vi "ADIS16470 IMU Example.vi"() -> ()   [LabVIEW 2019]
uses:
  <vilib>/Utility/RT CPU Load.ctl
  ADIS16470Lib/Typedef/ADIS16470 Hardware Configuration.ctl
  <vilib>/Rock Robotics/WPI/SPI/WPI_SPIMode.ctl
  <vilib>/Rock Robotics/SystemInterfaces/DIO/FPGA_DIOChannel.ctl
  <vilib>/Rock Robotics/SystemInterfaces/spilib/spi_bus.ctl
  ADIS16470Lib/Typedef/ADIS16470 Calibration Time.ctl
  ADIS16470Lib/SubVI/ADIS16470 Globals.vi
  <vilib>/NI_Real-Time Target Support.lvlib
panel:
  out "DiagStat":u16
  out "TempDegC":dbl
  out "RegAccumData":dbl[](array[numeric])
  out "RawReadData":u16[](array[numeric])
  out "Loop State":i32
  in  "Use Register Read Mode":bool
  in  "Initial Calibration Time (4s)":T1=enum."4s"
  in  "Recalibrate?":bool
  in  "Reset?":bool
  out "Integrated Gyro Angle":T2(graph)
  out "Calibrated?":bool
  out "IMU Detected?":bool
  in  "Hardware Config":T3={"SPI Clock Rate (Hz)"=2000000.0, "IMU SPI Mode (3)"=enum."Mode 3 (Clk Idle High,Sample on Trailing)", "IMU Reset Pin"=enum."SPI Port CS2", "IMU SPI Bus"=enum."SPI On-Board, CS0", "IMU Data Ready Pin"=enum."SPI Port CS1", "Stall Config"={"Pow2BytesPerRead"=1, "StallTicks"=1000, "CsToSclkTicks"=5}}
  out "CPU loads":T7[](array[typedef]) {"ISR (%)" format="%#.2f"; "Idle (%)" format="%#.2f"; "Background (%)" format="%#.2f"; "Normal (%)" format="%#.2f"; "Above Normal (%)" format="%#.2f"; "High (%)" format="%#.2g"; "Timed Structures (%)" format="%#.2g"; "Time Critical (%)" format="%#.2g"; "Total (%)" format="%#.2g"}
  in  "stop":bool
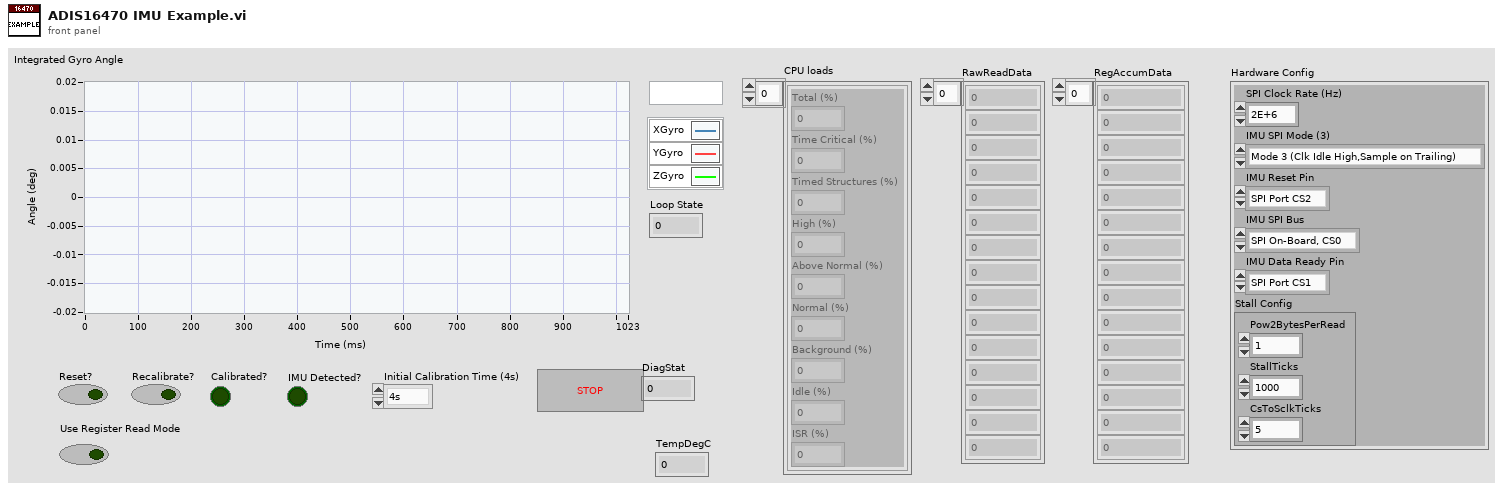
[diagram p1: front panel]
types:
  T1 = typedef "ADIS16470 Calibration Time.ctl" = enum16{"32ms", "64ms", "128ms", "256ms", "512ms", "1s", "2s", "4s", "8s", "16s", "32s", "64s"}
  T2 = cluster{"XAngle":dbl, "YAngle":dbl, "ZAngle":dbl}
  T3 = typedef "ADIS16470 Hardware Configuration.ctl" = cluster{"SPI Clock Rate (Hz)":dbl, "IMU SPI Mode (3)":T4, "IMU Reset Pin":T5, "IMU SPI Bus":T6, "IMU Data Ready Pin":T5, "Stall Config":cluster{"Pow2BytesPerRead":u8, "StallTicks":u16, "CsToSclkTicks":u8}}
  T4 = typedef "WPI_SPIMode.ctl" = enum16{"Mode 0 (Clk Idle Low,Sample on Leading)", "Mode 1 (Clk Idle Low,Sample on Trailing)", "Mode 2 (Clk Idle High,Sample on Leading)", "Mode 3 (Clk Idle High,Sample on Trailing)"}
  T5 = typedef "FPGA_DIOChannel.ctl" = enum8{"DIO 0", "DIO 1", "DIO 2", "DIO 3", "DIO 4", "DIO 5", "DIO 6", "DIO 7", "DIO 8", "DIO 9", "DIO MXP 0", "DIO MXP 1", "DIO MXP 2", "DIO MXP 3", "DIO MXP 4", "DIO MXP 5", "DIO MXP 6", "DIO MXP 7", "DIO MXP 8", "DIO MXP 9", "DIO MXP 10", "DIO MXP 11", "DIO MXP 12", "DIO MXP 13", "DIO MXP 14", "DIO MXP 15", "SPI Port CS1", "SPI Port CS2", "SPI Port CS3", "SPI Port MISO", "SPI Port MOSI", "Invalid"}
  T6 = typedef "spi_bus.ctl" = enum16{"SPI On-Board, CS0", "SPI On-Board, CS1", "SPI On-Board, CS2", "SPI On-Board, CS3", "SPI MXP", "Invalid"}
  T7 = typedef "NI_Real-Time Target Support.lvlib/RT CPU Load.ctl" = cluster{"Total (%)":dbl, "Time Critical (%)":dbl, "Timed Structures (%)":dbl, "High (%)":dbl, "Above Normal (%)":dbl, "Normal (%)":dbl, "Background (%)":dbl, "Idle (%)":dbl, "ISR (%)":dbl}
  T8 = typedef "ADIS16470 Device Reference.ctl" = cluster{"DevStatus":errorcluster, "Hardware Config":T3, "Calibration Complete":refnum<notifier>, "Status FIFO":refnum<k33>, "Last Value Reference":refnum<data-value>, "Sychronous Process VI":T9, "Cmd FIFO":refnum<k33>, "Source":T10, "Data FIFO":refnum<k33>, "Calibration Time":T1}
  T9 = typedef "ADIS16470 Process.ctl" = refnum<vi>
  T10 = typedef "FPGA_CounterEncoderSourceConvertionLVSourceType.ctl" = cluster{"DevStatus":errorcluster, "AnalogTriggerMode?":bool, "DigitalMode":cluster{"DIO Channel":T11}, "AnalogTriggerMode":cluster{"AnalogTriggerIndex":T12, "OutputType":T13}}
  T11 = typedef "FPGA_DIODigitalSourceChannel.ctl" = enum8{"DIO 0", "DIO 1", "DIO 2", "DIO 3", "DIO 4", "DIO 5", "DIO 6", "DIO 7", "DIO 8", "DIO 9", "DIO MXP 0", "DIO MXP 1", "DIO MXP 2", "DIO MXP 3", "DIO MXP 4", "DIO MXP 5", "DIO MXP 6", "DIO MXP 7", "DIO MXP 8", "DIO MXP 9", "DIO MXP 10", "DIO MXP 11", "DIO MXP 12", "DIO MXP 13", "DIO MXP 14", "DIO MXP 15", "SPI Port CS1", "SPI Port CS2", "SPI Port CS3", "SPI Port MISO", "SPI Port MOSI", "Disabled"}
  T12 = typedef "FPGA_AnalogTriggerIndex.ctl" = enum8{"Trig 0", "Trig 1", "Trig 2", "Trig 3", "Trig 4", "Trig 5", "Trig 6", "Trig 7", "Invalid"}
  T13 = typedef "FPGA_AnalogTriggerOutType.ctl" = enum16{"InWindow", "TriggerState", "Rising", "Falling"}
  T14 = typedef "ADIS16470 Status.ctl" = cluster{"Calibrated?":bool, "IMU Detected?":bool}
  T15 = typedef "ADIS16470 Data.ctl" = cluster{"XAngle":dbl, "YAngle":dbl, "ZAngle":dbl}
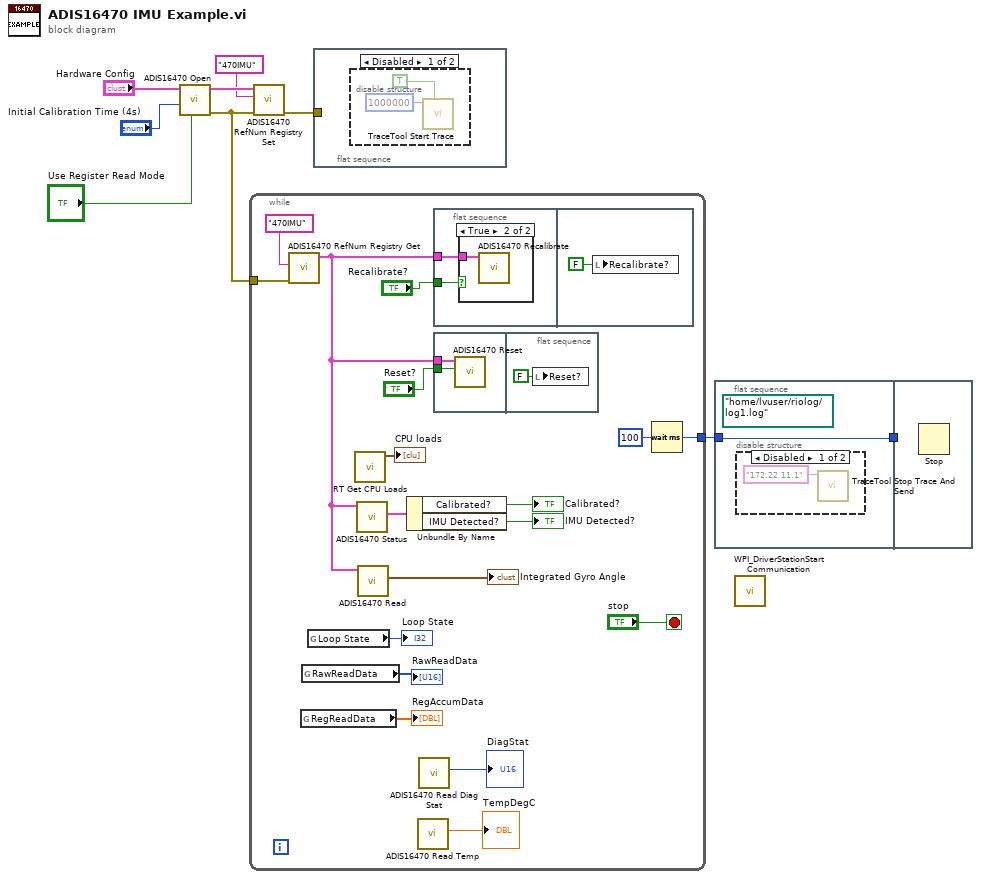
[diagram p0: block diagram]
diagram:
  n1 = call "ADIS16470 Open.vi"("Use Register Read Mode"="Use Register Read Mode", "Initial Calibration Time (4s)"="Initial Calibration Time (4s)", "Hardware Config"="Hardware Config") -> ("error out"=w2:errorcluster, "ADIS16470DevRef"=w4:T8)  [unwired: 7 in]
  n2 = while {
    tunnel: [w24] -> w9
    tunnel: w2 -> [w17]
    stop <- "stop" stop-if-true
    n3 = call "ADIS16470 RefNum Registry Get.vi"("error in (no error)"=w17, "refnum name"="470IMU") -> ("ADIS16470DevRef out"=w15:T8)  [unwired: 8 in, 1 out]
    n4 = global read "ADIS16470 Globals.vi" "RegReadData"() -> (→"RegAccumData":dbl[])
    n5 = global read "ADIS16470 Globals.vi" "RawReadData"() -> (→"RawReadData":u16[])
    n6 = global read "ADIS16470 Globals.vi" "Loop State"() -> (→"Loop State":i32)
    n7 = call <vilib>:"RT Get CPU Loads.vi"() -> ("CPU loads"=→"CPU loads":T7[])  [unwired: 10 in, 1 out]
    n8 = call "ADIS16470 Status.vi"("ADIS16470DevRef"=w15) -> ("ADIS16470 Status"=w22:T14)  [unwired: 8 in, 2 out]
    n9 = call "ADIS16470 Read.vi"("ADIS16470DevRef"=w15) -> ("ADIS16470 Value"=→"Integrated Gyro Angle":T15)  [unwired: 7 in, 3 out]
    n10 = Unbundle By Name(w22) -> ("Calibrated?"=→"Calibrated?":bool, "IMU Detected?"=→"IMU Detected?":bool)
    n11 = call "ADIS16470 Read Temp.vi"() -> ("TempDegC"=→"TempDegC":dbl)  [unwired: 9 in, 2 out]
    n12 = call "ADIS16470 Read Diag Stat.vi"() -> ("DiagStat"=→"DiagStat":u16)  [unwired: 9 in, 2 out]
    n13 = flat-sequence {
      tunnel: "Recalibrate?" -> [w28]
      tunnel: w15 -> [w29]
      frame #0 {
        n14 = case shown="True" w28 {
          tunnel: w29 -> [_ w30]
          frame False {
          }
          frame True {
            n15 = call "ADIS16470 Recalibrate.vi"("ADIS16470DevRef in"=w30) -> ()  [unwired: 9 in, 2 out]
          }
        }
      }
      frame #1 {
        n16 = local write "Recalibrate?"(FALSE ("Recalibrate?")) -> ()
      }
    }
    n17 = flat-sequence {
      tunnel: "Reset?" -> [w33]
      tunnel: w15 -> [w32]
      frame #0 {
        n18 = call "ADIS16470 Reset.vi"("Reset?"=w33, "ADIS16470DevRef"=w32) -> ()  [unwired: 8 in, 2 out]
      }
      frame #1 {
        n19 = local write "Reset?"(FALSE ("Reset?")) -> ()
      }
    }
    n20 = Wait (ms)(milliseconds to wait=u32 100) -> (millisecond timer value=w24:u32)
  }
  n21 = call "ADIS16470 RefNum Registry Set.vi"("error in (no error)"=w2, "refnum name"="470IMU", "ADIS16470DevRef in"=w4) -> ("error out"=w5:errorcluster)  [unwired: 7 in, 1 out]
  n22 = flat-sequence {
    tunnel: w5 -> [_]
    frame #0 {
      n23 = disable-structure shown="Disabled" {
        frame Disabled {
          n24 = call <vilib>:"TraceTool Start Trace.vi"("Detailed Tracing? (F)"=TRUE, "Buffer Size (250000 bytes)"=1000000) -> ()  [unwired: 8 in, 2 out]
        }
        frame Enabled {
        }
      }
    }
  }
  n25 = flat-sequence {
    tunnel: w9 -> [w37]
    tunnel: [w37] -> w7
    tunnel: w7 -> [_]
    frame #0 {
      (unwired) path "/home/lvuser/riolog/log1.log" ("Path to Trace Log")
      n26 = disable-structure shown="Disabled" {
        frame Disabled {
          n27 = call <vilib>:"TraceTool Stop Trace And Send.vi"("Trace Host Network Address"="172.22.11.1") -> ()  [unwired: 10 in, 1 out]
        }
        frame Enabled {
        }
      }
    }
    frame #1 {
      n28 = Stop() -> ()  [unwired: 1 in]
    }
  }
  n29 = call <vilib>:"WPI_DriverStationStart Communication.vi"() -> ()  [unwired: 12 in]
